vi "actuate.vi"(0 "IActuator in":refnum<class "IActuator.lvclass">, 5 "ILC in":refnum<class "ILC.lvclass">, 7 "Actuate Settings":T1, 11 "error in (no error)":errorcluster) -> (4 "IActuator out":refnum<class "IActuator.lvclass">, 6 "ILC out":refnum<class "ILC.lvclass">, 15 "error out":errorcluster)   [LabVIEW 2015, in "IActuator.lvclass"]
uses:
  IActuator.lvclass
  <userlib>/Common/ILC/ILC/ILC.lvclass
  Typedefs/Actuate Settings.ctl
  Typedefs/ControlMode.ctl
  Typedefs/FAMTTypedefs.lvlib
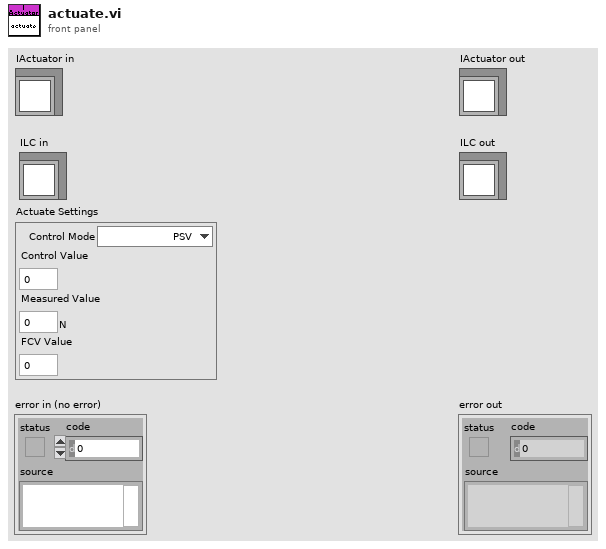
[diagram p1: front panel]
types:
  T1 = typedef "FAMTTypedefs.lvlib/Actuate Settings.ctl" = cluster{"Control Mode":T2, "Control Value":dbl, "Measured Value":dbl[unit], "FCV Value":dbl}
  T2 = typedef "FAMTTypedefs.lvlib/ControlMode.ctl" = enum16{"PSV", "FCV", "Both"}
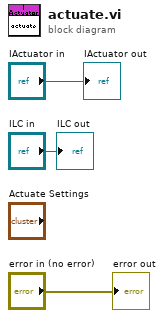
[diagram p0: block diagram]
diagram:
  "error out" <- "error in (no error)"
  "IActuator out" <- "IActuator in"
  "ILC out" <- "ILC in"
